vi "Input Type.vi"() -> (2 "Mode":i32)   [LabVIEW 2013]
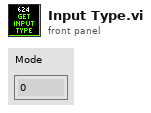
[diagram p1: front panel]
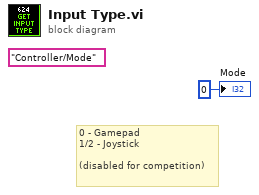
[diagram p0: block diagram]
diagram:
  (unwired) "Controller/Mode" ("Name")
  # "0 - Gamepad\n1/2 - Joystick\n\n(disabled for competition)"
  "Mode" <- 0 ("Mode")
